vi "UpdateAENames(SubVI).vi"(8 "error in (no error)":errorcluster, 10 "AE-NamesMapping":T1(array[cluster]), 11 "Data Value Reference In":refnum<data-value>) -> (0 "error out":errorcluster, 3 "Data Value Reference out":refnum<data-value>)   [LabVIEW 2017, in "DS_Lib.lvlib" / "SRReportParser.lvlib"]
uses:
  SRReportParser.lvlib
  Modules/Private Controls/Report Data Cluster.ctl
  Modules/Private Controls/Data Raw.ctl
  Modules/Data Operations.lvlib
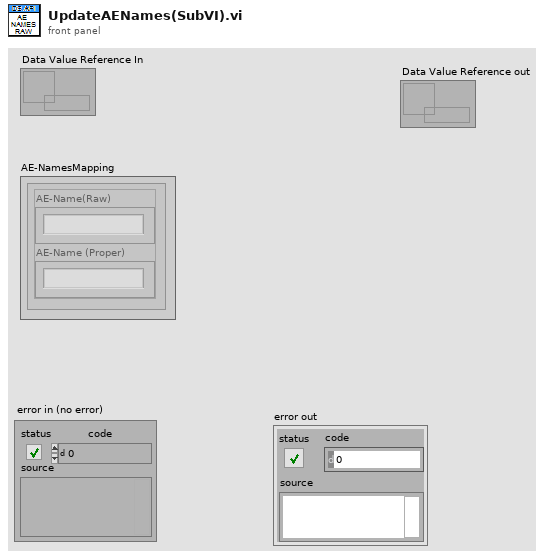
[diagram p1: front panel]
types:
  T1 = cluster{"AE-Name(Raw)":string, "AE-Name (Proper)":string}[]
  T2 = typedef "Data Operations.lvlib/Report Data Cluster.ctl" = cluster{"Headers":cluster{"Start Date":timestamp, "End Date":timestamp, "SR Status String":string[], "AE Owner String":string[]}, "Data":T3[]}
  T3 = typedef "Data Operations.lvlib/Data Raw.ctl" = cluster{"SR Number":string, "Status":string, "Summary":string, "AE Owner":string, "AE Group":string, "Contact":string, "SurveyData":cluster{"Resolution Time":dbl, "Total Satisfaction":dbl, "Response Time":dbl, "Courtesy":dbl, "Problem Solved":dbl, "Level of effort":dbl}, "Time Data":cluster{"Last Update Date":timestamp, "Creation Date":timestamp, "Creation week":i16, "Last Update Week":i16, "Creation Year":i16}}
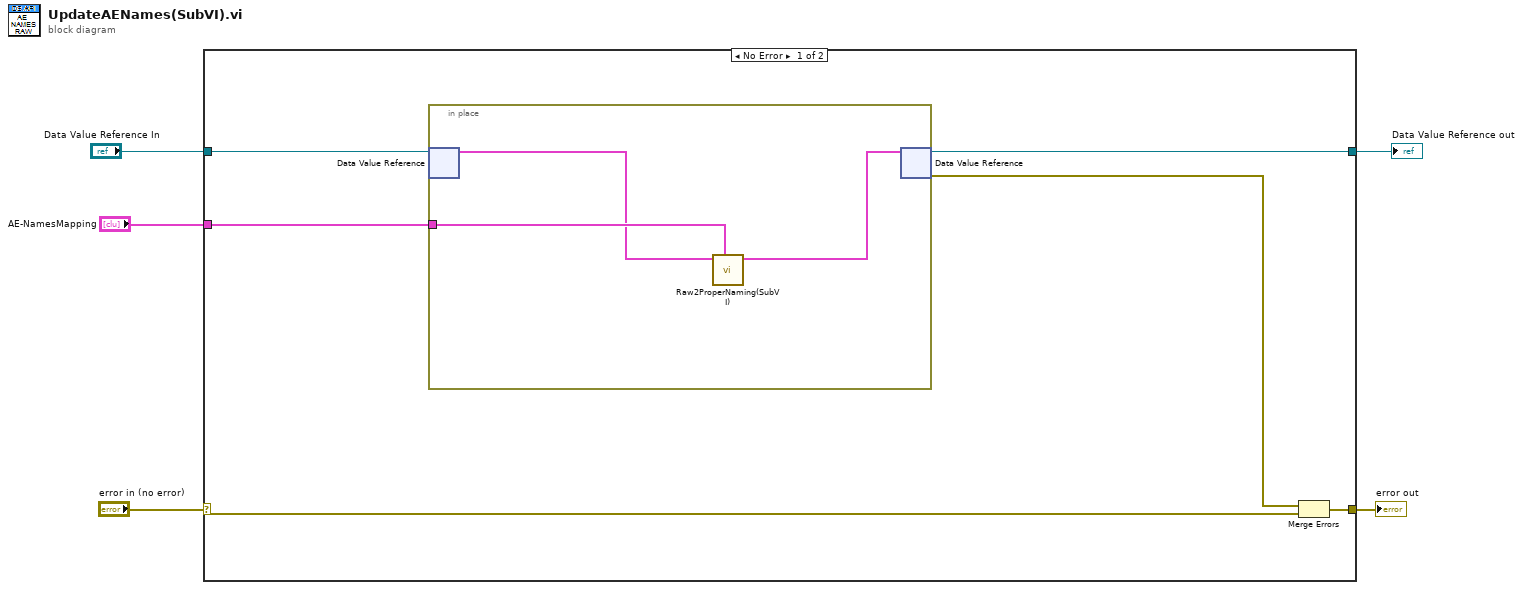
[diagram p0: block diagram]
diagram:
  n1 = case shown="No Error" "error in (no error)" {
    selector: "error in (no error)" -> [w9 w16]
    tunnel: [w10 w16] -> w5
    tunnel: [w8 w15] -> w1
    tunnel: "AE-NamesMapping" -> [w7 _]
    tunnel: "Data Value Reference In" -> [w6 w15]
    frame No Error {
      n2 = in-place {
        in-place-border: w7 -> [w14]
        n3 = in-place-dvr #1(w6) -> (w12:T2)  [unwired: 1 out]
        n4 = call "Raw2ProperNaming(SubVI).vi"("AE-NamesMapping"=w14, "Report Data"=w12) -> ("Report Data out"=w13:T2)  [unwired: 9 in]
        n5 = in-place-dvr #1(w13) -> (w8:refnum<data-value>, w11:errorcluster)
      }
      n6 = Merge Errors(w11, w9) -> (w10:errorcluster)
    }
    frame Error {
    }
  }
  "error out" <- w5
  "Data Value Reference out" <- w1
